vi "plot_add.vi"(5 "Input Points":dbl[](array[numeric])=[0.0, 0.0, 0.0], 9 "Input Arrays":dbl[][](array[numeric])=[[1.0, 4.0, 7.0], [2.0, 5.0, 8.0], [3.0, 6.0, 9.0]]) -> (10 "Output Arrays":dbl[][](array[numeric]), 13 "Timestamps":dbl[](array[numeric]))   [LabVIEW 2018]
doc: "Adds the datapoints for Timestamp, Rain Rate, and Accumulation to their corresponding plot arrays."
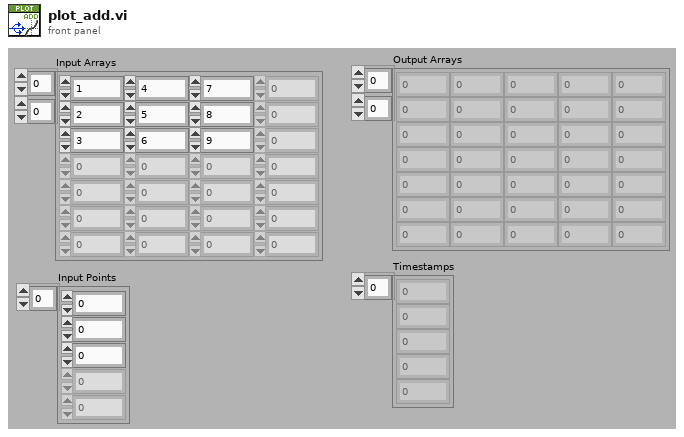
[diagram p1: front panel]
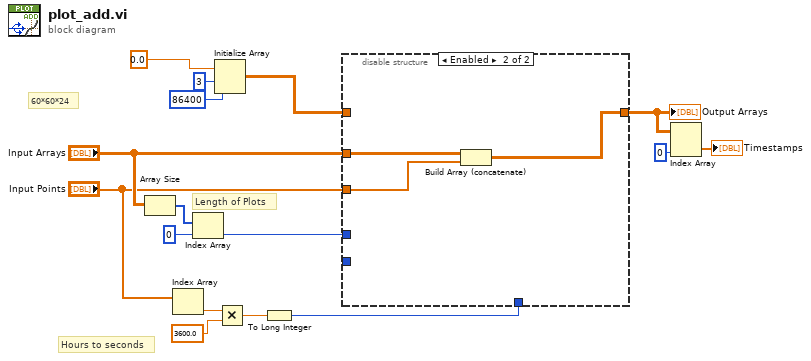
[diagram p0: block diagram]
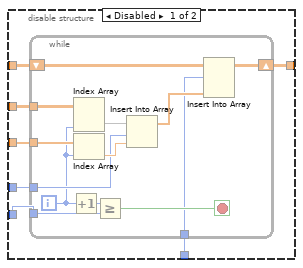
[diagram p2: hidden frame]
diagram:
  # "Hours to seconds"
  # "60*60*24"
  # "Length of Plots"
  n1 = Array Size(array="Input Arrays") -> (size(s)=w16:i32[])
  n2 = Index Array(array="Input Points") -> (element=w4:dbl)  [unwired: 1 in]
  n3 = Index Array(array=w16, index=0) -> (element=w15:i32)
  n4 = Initialize Array(0.0 ("Point H"), 3 ("dimension size"), 86400 ("dimension size")) -> (w9:dbl[][])
  n5 = Multiply(x=w4, y=3600.0) -> (x*y=w2:dbl)
  n6 = To Long Integer(number=w2) -> (32bit integer=w1:i32)
  n7 = disable-structure shown="Enabled" {
    disable-tunnel: w15 -> [w23 _]
    disable-tunnel: "Input Arrays" -> [w22 w39]
    disable-tunnel: [w21 w38] -> w12
    disable-tunnel: _ -> [w20 _]
    disable-tunnel: w9 -> [w19 _]
    disable-tunnel: "Input Points" -> [w18 w37]
    disable-tunnel: w1 -> [w17 _]
    frame Disabled {
      n8 = while {
        tunnel: w20 -> [w28]
        tunnel: w23 -> [w29]
        tunnel: w22 -> [w36]
        tunnel: w18 -> [w35]
        shift-right: [w34] -> w21
        shift-left: w19 -> [w32]
        tunnel: w17 -> [w24]
        i -> [w25]
        stop <- w27 stop-if-true
        n9 = Increment(x=w25) -> (x+1=w26:i32)
        n10 = Index Array(array=w36, index (col)=w25) -> (element=w31:dbl[])  [unwired: 1 in]
        n11 = Index Array(array=w35, index=w25) -> (element=w30:dbl)
        n12 = Greater Or Equal?(x=w26, y=w28) -> (x >= y?=w27:bool)
        n13 = Insert Into Array(array=w31, index=w29, new element=w30) -> (w33:dbl[])
        n14 = Insert Into Array(array=w32, index (row)=w24, new element=w33) -> (w34:dbl[][])  [unwired: 1 in]
      }
    }
    frame Enabled {
      n15 = Build Array (concatenate)(w39, w37) -> (w38:dbl[][])
    }
  }
  "Output Arrays" <- w12
  n16 = Index Array(array=w12, index (col)=0 ("disabled index (col)")) -> (element=→"Timestamps":dbl[])  [unwired: 1 in]
